vi "example-write-read-image.vi"() -> ()   [LabVIEW 2023]
uses:
  gfitsio.lvlib
  cfitsio-bitpix.ctl
panel:
  out "Primary Array\nData Match\n(variant read)":bool
  out "Primary Array\nData Match\n(1D read)":bool
  out "Primary Array\nData Match\n(scalar read)":bool
  out "Image Extension\nData Array":i32[][][](array[numeric])
  out "Primary Image\nData Array":i32[][][](array[numeric])
  out "error out":errorcluster
  # "page"
  # "row"
  # "column"
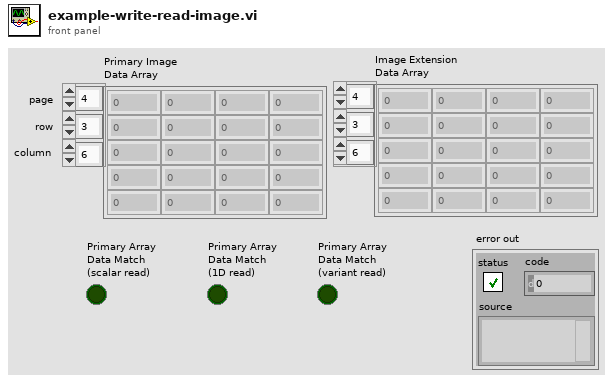
[diagram p1: front panel]
types:
  T1 = enum16{"open", "open or create", "create or replace", "create", "open (read only)"}
  T2 = typedef "gfitsio.lvlib/cfitsio-bitpix.ctl" = i32
  T3 = typedef "gfitsio.lvlib/gfitsio-refnum.ctl" = refnum<k1>
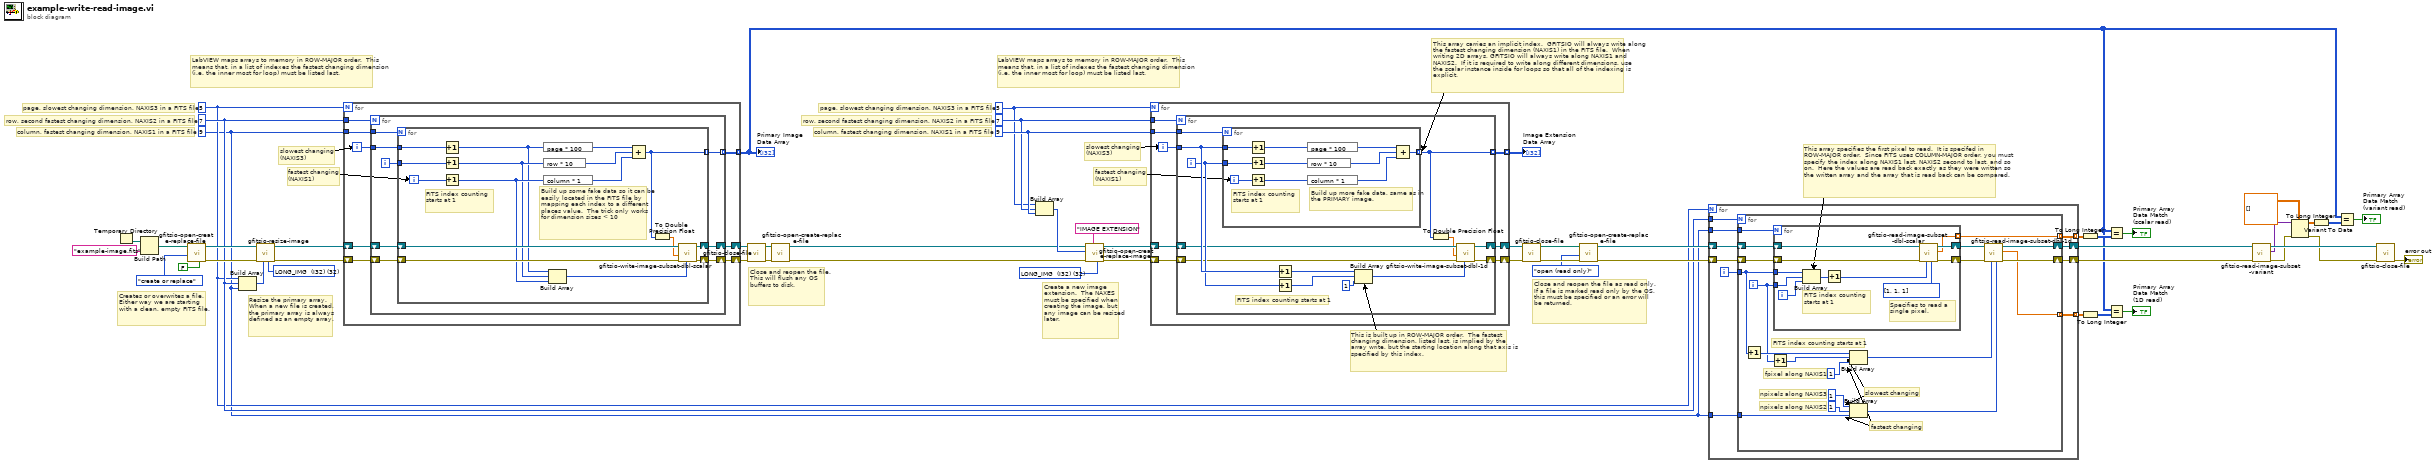
[diagram p0: block diagram]
diagram:
  w36 = 5
  w37 = 7
  w38 = 9
  w29 = T2 32 items=["<invalid type>"=0, "BYTE_IMG  (U8)"=8, "SHORT_IMG  (I16)"=16, "USHORT_IMG  (U16)"=20, "LONG_IMG  (I32)"=32, "ULONG_IMG  (U32)"=40, "FLOAT_IMG  (SGL)"=-32, "DOUBLE_IMG  (DBL)"=-64] ("image data type")
  w19 = 5
  w20 = 7
  w15 = 9
  w48 = T2 32 items=["<invalid type>"=0, "BYTE_IMG  (U8)"=8, "SHORT_IMG  (I16)"=16, "USHORT_IMG  (U16)"=20, "LONG_IMG  (I32)"=32, "ULONG_IMG  (U32)"=40, "FLOAT_IMG  (SGL)"=-32, "DOUBLE_IMG  (DBL)"=-64] ("image data type")
  # "This array specifies the first pixel to read.  It is specifed in ROW-MAJOR order.  Since FITS uses COLUMN-MAJOR order, you must specify the index along NAXIS1 last, NAXIS2 second to last, and so on.  Here the values are read back exactly as they were written so the written array and the array that is read back can be compared."
  # "This is built up in ROW-MAJOR order.  The fastest changing dimension, listed last, is implied by the array write, but the starting location along that axis is specified by this index."
  # "This array carries an implicit index.  GFITSIO will always write along the fastest changing dimension (NAXIS1) in the FITS file.  When writing 2D arrays, GFITSIO will always write along NAXIS1 and NAXIS2.  If it is required to write along different dimensions, use the scalar instance inside for loops so that all of the indexing is explicit."
  # "Close and reopen the file as read only.  If a file is marked read only by the OS, this must be specified or an error will be returned."
  # "slowest changing\n(NAXIS3)"
  # "fastest changing\n(NAXIS1)"
  # "LabVIEW maps arrays to memory in ROW-MAJOR order.  This means that, in a list of indexes the fastest changing dimension (i.e. the inner most for loop) must be listed last."
  # "Create a new image extension.  The NAXES must be specified when creating the image, but any image can be resized later."
  # "page, slowest changing dimension, NAXIS3 in a FITS file"
  # "row, second fastest changing dimension, NAXIS2 in a FITS file"
  # "column, fastest changing dimension, NAXIS1 in a FITS file"
  # "Close and reopen the file.  This will flush any OS buffers to disk."
  # "Creates or overwrites a file.  Either way we are starting with a clean, empty FITS file."
  # "slowest changing\n(NAXIS3)"
  # "fastest changing\n(NAXIS1)"
  # "LabVIEW maps arrays to memory in ROW-MAJOR order.  This means that, in a list of indexes the fastest changing dimension (i.e. the inner most for loop) must be listed last."
  # "Resize the primary array.  When a new file is created, the primary array is always defined as an empty array."
  # "page, slowest changing dimension, NAXIS3 in a FITS file"
  # "row, second fastest changing dimension, NAXIS2 in a FITS file"
  # "column, fastest changing dimension, NAXIS1 in a FITS file"
  n1 = Temporary Directory() -> (w41:path)
  n2 = Build Path(base path=w41, name or relative path="example-image.fits") -> (appended path=w39:path)
  n3 = call "gfitsio-open-create-replace-file.vi"("advisory dialog? (display:T)"=FALSE, "function (open)"=T1."create or replace", "file path (dialog if empty)"=w39) -> ("error out"=w50:errorcluster, "gfits refnum"=w51:T3)  [unwired: 6 in, 1 out]
  n4 = Build Array(w19, w20, w15) -> (w47:i32[])
  n5 = call "gfitsio-resize-image.vi"("image data type"=w48, "naxes"=w47, "error in (no error)"=w50, "gfits refnum"=w51) -> ("error out"=w46:errorcluster, "dup gfits refnum"=w49:T3)  [unwired: 6 in]
  n6 = for {
    N: w19 -> [_]
    shift-right: [w60] -> w52
    shift-left: w49 -> [w61]
    tunnel: w20 -> [w59]
    tunnel: w15 -> [w58]
    shift-right: [w56] -> w45
    shift-left: w46 -> [w57]
    tunnel: [w55] -> w1 mode=indexing
    i -> [w62]
    n7 = for {
      N: w59 -> [_]
      tunnel: w62 -> [w69]
      shift-right: [w67] -> w60
      shift-left: w61 -> [w68]
      tunnel: w58 -> [w66]
      shift-right: [w64] -> w56
      shift-left: w57 -> [w65]
      tunnel: [w63] -> w55 mode=indexing
      i -> [w70]
      n8 = for {
        N: w66 -> [_]
        tunnel: w70 -> [w85]
        tunnel: w69 -> [w86]
        shift-right: [w82] -> w67
        shift-left: w68 -> [w83]
        shift-right: [w75] -> w64
        shift-left: w65 -> [w76]
        tunnel: [w71] -> w63 mode=indexing
        i -> [w84]
        # "Build up some fake data so it can be easily located in the FITS file by mapping each index to a different places value.  The trick only works for dimension sizes < 10"
        # "FITS index counting starts at 1"
        n9 = Increment(x=w86) -> (x+1=w72:i32)
        n10 = Increment(x=w85) -> (x+1=w73:i32)
        n11 = Increment(x=w84) -> (x+1=w74:i32)
        n12 = expression code="page * 100"(w72) -> (w81:i32)
        n13 = expression code="row * 10"(w73) -> (w80:i32)
        n14 = expression code="column * 1"(w74) -> (w79:i32)
        n15 = Build Array(w72, w73, w74) -> (w78:i32[])
        n16 = Compound Arithmetic op=ADD(w81, w80, w79) -> (w71:i32)
        n17 = To Double Precision Float(number=w71) -> (double precision float=w77:dbl)
        n18 = call "gfitsio-write-image-subset-dbl-scalar.vi"("fpixel"=w78, "error in (no error)"=w76, "data"=w77, "gfits refnum"=w83) -> ("error out"=w75:errorcluster, "dup gfits refnum"=w82:T3)  [unwired: 6 in]
      }
    }
  }
  "Primary Image\nData Array" <- w1
  n19 = call "gfitsio-close-file.vi"("error in (no error)"=w45, "gfits refnum"=w52) -> ("error out"=w44:errorcluster, "Path"=w42:path)  [unwired: 8 in]
  n20 = call "gfitsio-open-create-replace-file.vi"("error in (no error)"=w44, "file path (dialog if empty)"=w42) -> ("error out"=w25:errorcluster, "gfits refnum"=w26:T3)  [unwired: 7 in, 1 out]
  n21 = Build Array(w36, w37, w38) -> (w30:i32[])
  n22 = call "gfitsio-open-create-replace-image.vi"("image data type"=w29, "hdu name (dialog if empty)"="IMAGE EXTENSION", "error in (no error)"=w25, "naxes"=w30, "gfits refnum"=w26) -> ("error out"=w31:errorcluster, "dup gfits refnum"=w28:T3)  [unwired: 4 in, 1 out]
  n23 = for {
    N: w36 -> [_]
    shift-right: [w92] -> w27
    shift-left: w28 -> [w93]
    tunnel: w37 -> [w91]
    tunnel: w38 -> [w90]
    shift-right: [w88] -> w32
    shift-left: w31 -> [w89]
    tunnel: [w87] -> w33 mode=indexing
    i -> [w94]
    n24 = for {
      N: w91 -> [_]
      tunnel: w94 -> [w106]
      shift-right: [w101] -> w92
      shift-left: w93 -> [w103]
      tunnel: w90 -> [w97]
      shift-right: [w100] -> w88
      shift-left: w89 -> [w102]
      tunnel: [w107] -> w87 mode=indexing
      i -> [w105]
      # "FITS index counting starts at 1"
      n25 = for {
        N: w97 -> [_]
        tunnel: w105 -> [w117]
        tunnel: w106 -> [w116]
        tunnel: [w115] -> w107 mode=indexing
        i -> [w108]
        # "Build up more fake data, same as in the PRIMARY image."
        # "FITS index counting starts at 1"
        n26 = Increment(x=w116) -> (x+1=w109:i32)
        n27 = Increment(x=w117) -> (x+1=w110:i32)
        n28 = Increment(x=w108) -> (x+1=w111:i32)
        n29 = expression code="page * 100"(w109) -> (w114:i32)
        n30 = expression code="row * 10"(w110) -> (w113:i32)
        n31 = expression code="column * 1"(w111) -> (w112:i32)
        n32 = Compound Arithmetic op=ADD(w114, w113, w112) -> (w115:i32)
      }
      n33 = Increment(x=w106) -> (x+1=w96:i32)
      n34 = Increment(x=w105) -> (x+1=w95:i32)
      n35 = Build Array(w96, w95, 1 ("element")) -> (w99:i32[])
      n36 = To Double Precision Float(number=w107) -> (double precision float=w98:dbl[])
      n37 = call "gfitsio-write-image-subset-dbl-1d.vi"("fpixel"=w99, "error in (no error)"=w102, "data"=w98, "gfits refnum"=w103) -> ("error out"=w100:errorcluster, "dup gfits refnum"=w101:T3)  [unwired: 6 in]
    }
  }
  "Image Extension\nData Array" <- w33
  n38 = call "gfitsio-close-file.vi"("error in (no error)"=w32, "gfits refnum"=w27) -> ("error out"=w34:errorcluster, "Path"=w35:path)  [unwired: 8 in]
  n39 = call "gfitsio-open-create-replace-file.vi"("error in (no error)"=w34, "function (open)"=T1."open (read only)", "file path (dialog if empty)"=w35) -> ("error out"=w21:errorcluster, "gfits refnum"=w22:T3)  [unwired: 6 in, 1 out]
  n40 = for {
    N: w19 -> [_]
    shift-right: [w126] -> w11
    shift-left: w21 -> [w127]
    shift-right: [w124] -> w10
    shift-left: w22 -> [w125]
    tunnel: w15 -> [w123]
    tunnel: w20 -> [w122]
    tunnel: [w120] -> w18 mode=indexing
    tunnel: w15 -> [w119]
    tunnel: [w118] -> w12 mode=indexing
    i -> [w121]
    n41 = for {
      N: w122 -> [_]
      shift-right: [w139] -> w126
      shift-left: w127 -> [w146]
      shift-right: [w140] -> w124
      shift-left: w125 -> [w145]
      tunnel: w123 -> [w144]
      tunnel: w121 -> [w131]
      tunnel: [w143] -> w120 mode=indexing
      tunnel: w119 -> [w138]
      tunnel: [w134] -> w118 mode=indexing
      i -> [w129]
      # "fastest changing"
      # "slowest changing"
      # "fpixel along NAXIS1"
      # "npixels along NAXIS2"
      # "npixels along NAXIS3"
      # "FITS index counting starts at 1"
      n42 = Increment(x=w131) -> (x+1=w130:i32)
      n43 = Increment(x=w129) -> (x+1=w128:i32)
      n44 = for {
        N: w144 -> [_]
        shift-right: [w156] -> w142
        shift-left: w146 -> [w157]
        shift-right: [w154] -> w141
        shift-left: w145 -> [w155]
        tunnel: w129 -> [w149]
        tunnel: w131 -> [w148]
        tunnel: [w147] -> w143 mode=indexing
        i -> [w150]
        # "Specifies to read a single pixel."
        # "FITS index counting starts at 1"
        n45 = Build Array(w148, w149, w150) -> (w152:i32[])
        n46 = Increment(x=w152) -> (x+1=w151:i32[])
        n47 = call "gfitsio-read-image-subset-dbl-scalar.vi"("npixels (rest)"=i32[] [1, 1, 1], "fpixel (origin)"=w151, "error in (no error)"=w157, "gfits refnum"=w155) -> ("error out"=w156:errorcluster, "data"=w147:dbl, "dup gfits refnum"=w154:T3)  [unwired: 5 in]
      }
      n48 = Build Array(w130, w128, 1 ("element")) -> (w132:i32[])
      n49 = Build Array(1 ("element"), 1 ("element"), w138) -> (w133:i32[])
      n50 = call "gfitsio-read-image-subset-dbl-1d.vi"("npixels (rest)"=w133, "fpixel (origin)"=w132, "error in (no error)"=w142, "gfits refnum"=w141) -> ("error out"=w139:errorcluster, "data"=w134:dbl[], "dup gfits refnum"=w140:T3)  [unwired: 5 in]
    }
  }
  n51 = To Long Integer(number=w18) -> (32bit integer=w17:i32[][][])
  n52 = To Long Integer(number=w12) -> (32bit integer=w13:i32[][][])
  n53 = Equal?(x=w1, y=w17) -> (x = y?=→"Primary Array\nData Match\n(scalar read)":bool)
  n54 = Equal?(x=w1, y=w13) -> (x = y?=→"Primary Array\nData Match\n(1D read)":bool)
  n55 = call "gfitsio-read-image-subset-variant.vi"("error in (no error)"=w11, "gfits refnum"=w10) -> ("error out"=w7:errorcluster, "Variant"=w8:variant, "dup gfits refnum"=w9:T3)  [unwired: 7 in]
  n56 = Variant To Data(error in=w7, type=dbl[][][] [] ("npixels (rest)"), Variant=w8) -> (data=w2:dbl[][][], error out=w6:errorcluster)
  n57 = To Long Integer(number=w2) -> (32bit integer=w4:i32[][][])
  n58 = Equal?(x=w1, y=w4) -> (x = y?=→"Primary Array\nData Match\n(variant read)":bool)
  n59 = call "gfitsio-close-file.vi"("error in (no error)"=w6, "gfits refnum"=w9) -> ("error out"=→"error out":errorcluster)  [unwired: 8 in, 1 out]
